vi "HelioLED.vi"() -> ()   [LabVIEW 2010]
uses:
  bricks/classes/DAQmxDigitalOut/DAQmxDigitalOut.lvclass
  bricks/classes/DAQmxAnalogOut/DAQmxAnalogOut/DAQmxAnalogOut.lvclass
panel:
  in  "period":dbl[unit]=20.0
  in  "startButton":bool
  in  "number of points":i32=1 min=1
  out "lower bound":dbl[unit]
  out "upper bound":dbl[unit]
  in  "setUpperBoundButton":bool
  in  "setLowerBoundButton":bool
  in  "doneButton":bool
  in  "voltage":dbl[unit](slide) scale=0.0..4.0
  in  "voltage source configuration":string(combo)
  in  "trigger configuration":string(combo)
  # "HelioLED"
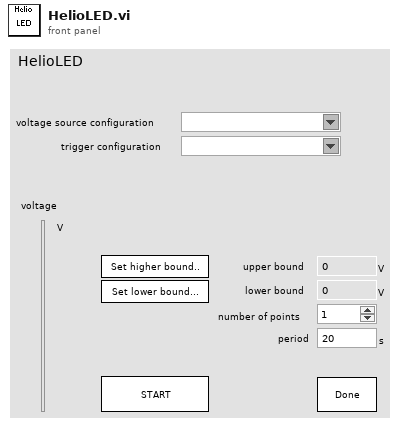
[diagram p1: front panel]
types:
  T1 = enum8{"Enabled", "Disabled", "Disabled and Grayed Out"}
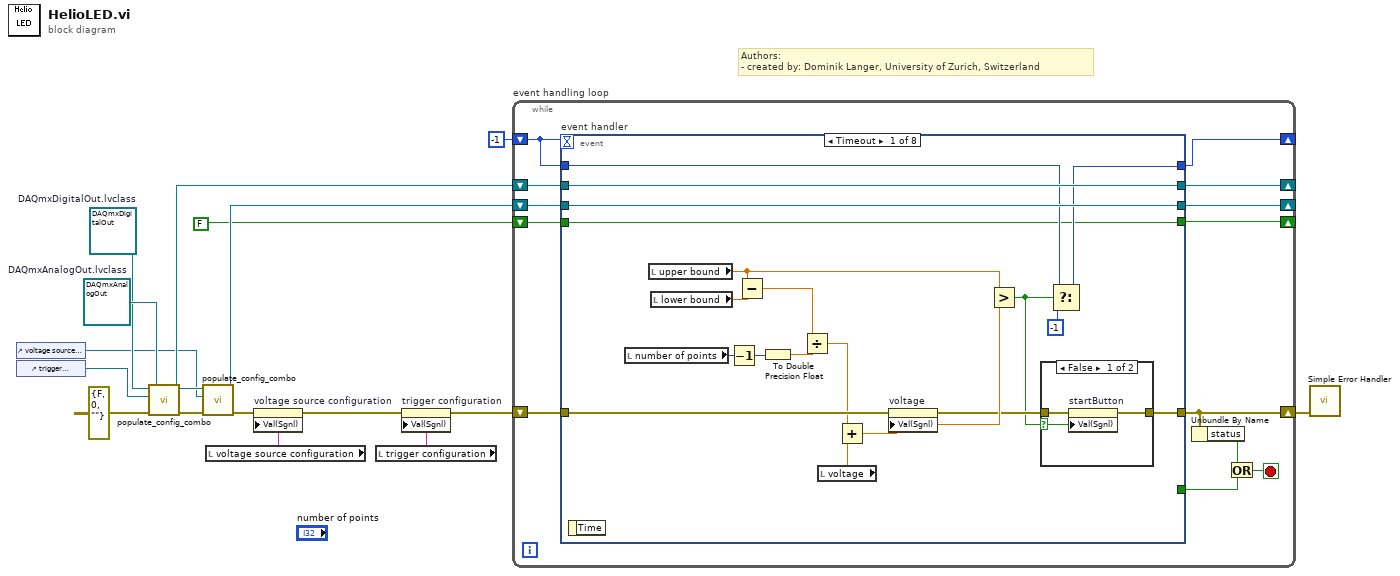
[diagram p0: block diagram]
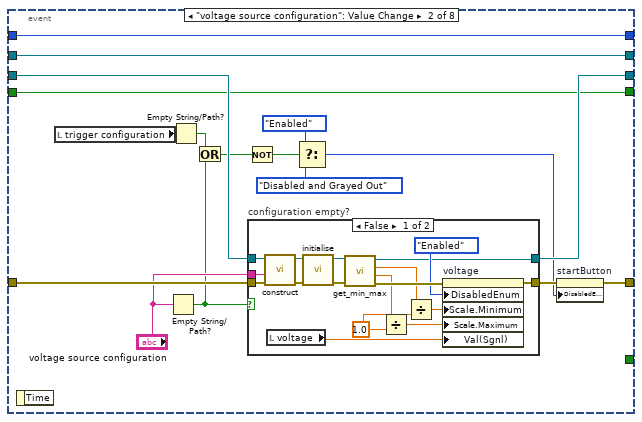
[diagram p3: hidden frame]
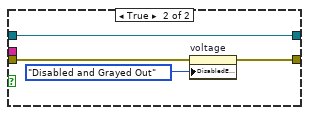
[diagram p4: hidden frame]
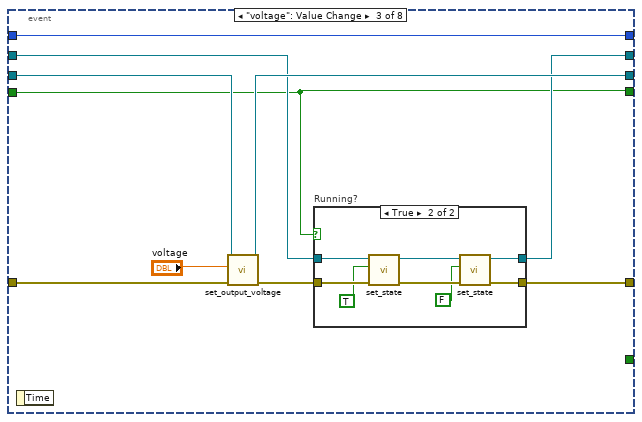
[diagram p5: hidden frame]
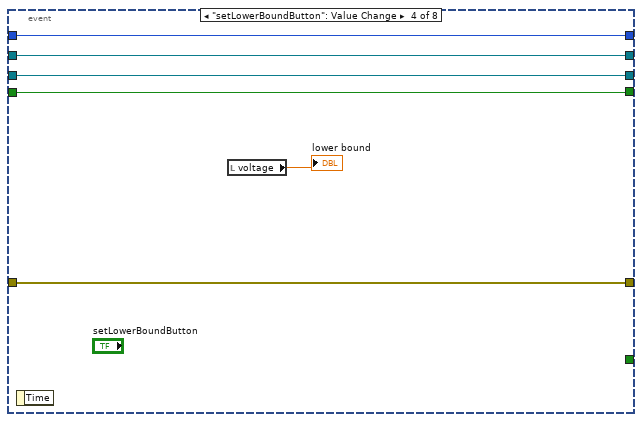
[diagram p7: hidden frame]
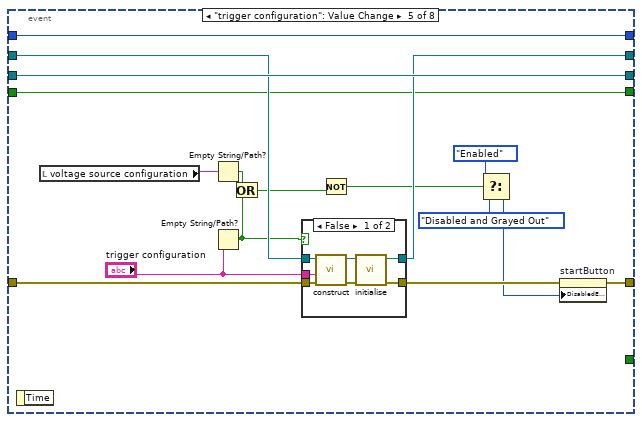
[diagram p8: hidden frame]
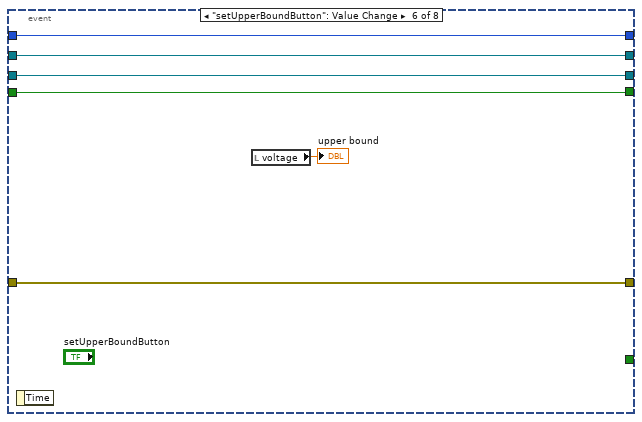
[diagram p10: hidden frame]
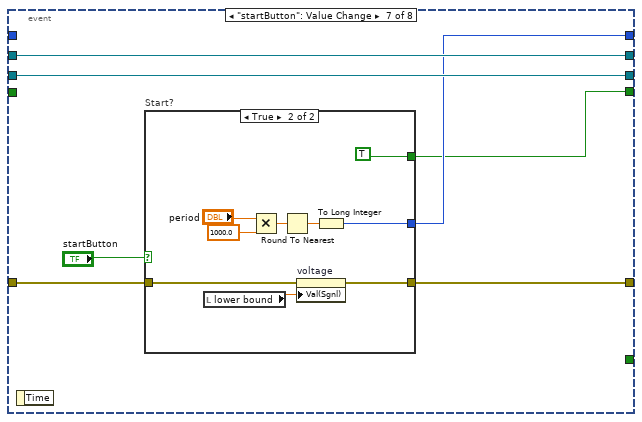
[diagram p11: hidden frame]
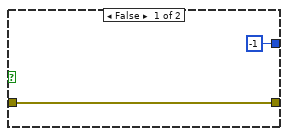
[diagram p12: hidden frame]
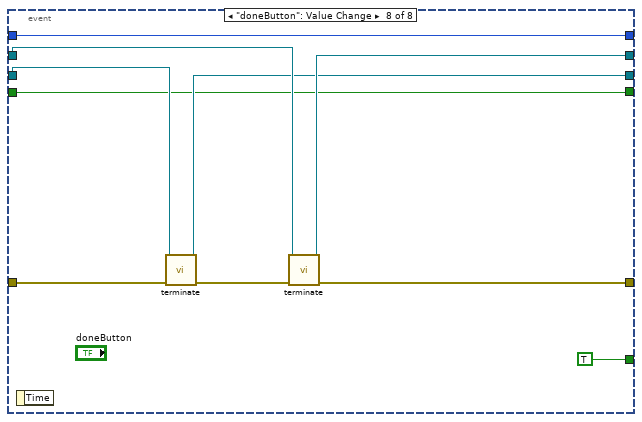
[diagram p13: hidden frame]
diagram:
  w14 = refnum<class "DAQmxAnalogOut.lvclass"> refnum  # DAQmxAnalogOut.lvclass
  w12 = refnum<class "DAQmxDigitalOut.lvclass"> refnum  # DAQmxDigitalOut.lvclass
  # "Authors: \n- created by: Dominik Langer, University of Zurich, Switzerland"
  n1 = control-ref of="voltage source configuration"() -> (w8:refnum<vi>)
  n2 = control-ref of="trigger configuration"() -> (w9:refnum<vi>)
  n3 = call-dynamic "populate_config_combo.vi"("error in (no error)"=errorcluster {"status"=FALSE, "code"=0, "source"=""}, "combo-box reference"=w9, "GenericPlugin in"=w12) -> ("error out"=w15:errorcluster, "GenericPlugin out"=w11:refnum<class "DAQmxDigitalOut.lvclass">)  [unwired: 7 in]
  n4 = call-dynamic "populate_config_combo.vi"("error in (no error)"=w15, "combo-box reference"=w8, "GenericPlugin in"=w14) -> ("error out"=w6:errorcluster, "GenericPlugin out"=w13:refnum<class "DAQmxAnalogOut.lvclass">)  [unwired: 7 in]
  n5 = local read "voltage source configuration"() -> (w3:string)
  n6 = property on="voltage source configuration" class="CmbBox"(error in=w6, "Val(Sgnl)"=w3) -> (error out=w5:errorcluster)  [unwired: 1 in, 1 out]
  n7 = local read "trigger configuration"() -> (w2:string)
  n8 = property on="trigger configuration" class="CmbBox"(error in=w5, "Val(Sgnl)"=w2) -> (error out=w4:errorcluster)  [unwired: 1 in, 1 out]
  n9 = while "event handling loop" {
    shift-right: [w28] -> _
    shift-left: -1 -> [w29]
    shift-right: [w26] -> w1
    shift-left: w4 -> [w27]
    shift-right: [w22] -> _
    shift-left: w11 -> [w20]
    shift-right: [w21] -> _
    shift-left: w13 -> [w19]
    shift-right: [w17] -> _
    shift-left: FALSE -> [w18]
    stop <- w23 stop-if-true
    n10 = event "event handler" shown="[0] Timeout" {
      selector: _ -> [_ _ _ _ _ _ _ _]
      dyn-events: _ -> [_ _ _ _ _ _ _ _]
      timeout: w29 -> [_ _ _ _ _ _ _ _]
      tunnel: [w34 w69 w100 w116 w133 w148 w153 w176] -> w28
      tunnel: w29 -> [w36 w69 w100 w116 w133 w148 _ w176]
      tunnel: w27 -> [w46 w67 w99 w115 w131 w147 w152 w169]
      tunnel: [w31 w59 w93 w115 w124 w147 w151 w168] -> w26
      tunnel: [_ _ _ _ _ _ _ TRUE] -> w25
      tunnel: [w48 w68 w92 w114 w129 w146 w155 w172] -> w22
      tunnel: [w47 w65 w96 w113 w132 w145 w154 w171] -> w21
      tunnel: w20 -> [w48 w68 w94 w114 w130 w146 w155 w173]
      tunnel: w19 -> [w47 w66 w97 w113 w132 w145 w154 w174]
      tunnel: [w33 w64 w91 w111 w128 w143 w150 w167] -> w17
      tunnel: w18 -> [w33 w64 w91 w111 w128 w143 _ w167]
      event Timeout {
        n11 = event-data() -> ()  [unwired: 1 in, 1 out]
        n12 = local read "number of points"() -> (w44:i32)
        n13 = local read "upper bound"() -> (w37:dbl[unit])
        n14 = local read "lower bound"() -> (w45:dbl[unit])
        n15 = Decrement(x=w44) -> (x-1=w43:i32)
        n16 = Subtract(x=w37, y=w45) -> (x-y=w42:dbl[unit])
        n17 = To Double Precision Float(number=w43) -> (double precision float=w41:dbl)
        n18 = Divide(x=w42, y=w41) -> (x/y=w39:dbl[unit])
        n19 = local read "voltage"() -> (w40:dbl[unit])
        n20 = Add(x=w39, y=w40) -> (x+y=w38:dbl[unit])
        n21 = property on="voltage" class="Slide (strict)"(error in=w46, "Val(Sgnl)"=w38) -> (error out=w32:errorcluster)  [unwired: 1 in, 1 out]
        n22 = Greater?(x=w37, y=w38) -> (0:w30:bool)
        n23 = case shown="False" w30 {
          selector: w30 -> [w49 _]
          tunnel: w32 -> [w51 w52]
          tunnel: [w50 w52] -> w31
          frame False {
            n24 = property on="startButton" class="Bool (strict)"(error in=w51, "Val(Sgnl)"=w49) -> (error out=w50:errorcluster)  [unwired: 1 in, 1 out]
          }
          frame True {
          }
        }
        n25 = Select(t=w36, s=w30, f=-1) -> (s? t:f=w34:i32)
      }
      event "voltage source configuration": Value Change {
        n26 = event-data() -> ()  [unwired: 1 in, 1 out]
        n27 = local read "trigger configuration"() -> (w62:string)
        n28 = Empty String/Path?(string/path="voltage source configuration") -> (empty?=w60:bool)
        n29 = Empty String/Path?(string/path=w62) -> (empty?=w61:bool)
        n30 = Or(x=w61, y=w60) -> (x .or. y?=w53:bool)
        n31 = Not(x=w53) -> (.not. x?=w54:bool)
        n32 = case "configuration empty?" shown="False" w60 {
          tunnel: w67 -> [w86 w89]
          tunnel: w66 -> [w85 w90]
          tunnel: [w81 w88] -> w58
          tunnel: [w71 w90] -> w65
          tunnel: "voltage source configuration" -> [w82 _]
          frame False {
            w72 = dbl[unit] 1.0 ("y")
            n33 = call-dynamic "construct.vi"("error in (no error)"=w86, "configuration name"=w82, "GenericPlugin in"=w85) -> ("error out"=w84:errorcluster, "GenericPlugin out"=w83:refnum<class "DAQmxAnalogOut.lvclass">)  [unwired: 7 in]
            n34 = local read "voltage"() -> (w70:dbl[unit])
            n35 = call-dynamic "initialise.vi"("error in (no error)"=w84, "DAQmxAnalogOut in"=w83) -> ("error out"=w80:errorcluster, "DAQmxAnalogOut out"=w79:refnum<class "DAQmxAnalogOut.lvclass">)  [unwired: 8 in]
            n36 = call "get_min_max.vi"("error in (no error)"=w80, "DAQmxAnalogOut.lvclass in"=w79) -> ("error out"=w78:errorcluster, "maximum"=w74:dbl[unit], "minimum"=w75:dbl[unit], "DAQmxAnalogOut.lvclass out"=w71:refnum<class "DAQmxAnalogOut.lvclass">)  [unwired: 6 in]
            n37 = Divide(x=w74, y=w72) -> (x/y=w73:dbl)
            n38 = Divide(x=w75, y=w72) -> (x/y=w76:dbl)
            n39 = property on="voltage" class="Slide (strict)"(error in=w78, "DisabledEnum"=T1."Enabled" ("Disabled"), "Scale.Minimum"=w76, "Scale.Maximum"=w73, "Val(Sgnl)"=w70) -> (error out=w81:errorcluster)  [unwired: 1 in, 1 out]
          }
          frame True {
            n40 = property on="voltage" class="Slide (strict)"(error in=w89, "DisabledEnum"=T1."Disabled and Grayed Out" ("Disabled")) -> (error out=w88:errorcluster)  [unwired: 1 in, 1 out]
          }
        }
        n41 = Select(t=T1."Enabled" ("Disabled"), s=w54, f=T1."Disabled and Grayed Out" ("Disabled")) -> (s? t:f=w55:T1)
        n42 = property on="startButton" class="Bool (strict)"(error in=w58, "DisabledEnum"=w55) -> (error out=w59:errorcluster)  [unwired: 1 in, 1 out]
      }
      event "voltage": Value Change {
        n43 = event-data() -> ()  [unwired: 1 in, 1 out]
        n44 = call "set_output_voltage.vi"("error in (no error)"=w99, "output value"="voltage", "DAQmxAnalogOut in"=w97) -> ("error out"=w95:errorcluster, "DAQmxAnalogOut out"=w96:refnum<class "DAQmxAnalogOut.lvclass">)  [unwired: 7 in]
        n45 = case "Running?" shown="True" w91 {
          tunnel: w95 -> [w101 w110]
          tunnel: w94 -> [w102 w109]
          tunnel: [w101 w106] -> w93
          tunnel: [w102 w104] -> w92
          frame False {
          }
          frame True {
            n46 = call "set_state.vi"("error in (no error)"=w110, "state"=TRUE, "DAQmxDigitalOut in"=w109) -> ("error out"=w107:errorcluster, "DAQmxDigitalOut out"=w105:refnum<class "DAQmxDigitalOut.lvclass">)  [unwired: 7 in]
            n47 = call "set_state.vi"("error in (no error)"=w107, "state"=FALSE, "DAQmxDigitalOut in"=w105) -> ("error out"=w106:errorcluster, "DAQmxDigitalOut out"=w104:refnum<class "DAQmxDigitalOut.lvclass">)  [unwired: 7 in]
          }
        }
      }
      event "setLowerBoundButton": Value Change {
        n48 = event-data() -> ()  [unwired: 1 in, 1 out]
        n49 = local read "voltage"() -> (→"lower bound":dbl[unit])
      }
      event "trigger configuration": Value Change {
        n50 = event-data() -> ()  [unwired: 1 in, 1 out]
        n51 = local read "voltage source configuration"() -> (w127:string)
        n52 = Empty String/Path?(string/path=w127) -> (empty?=w120:bool)
        n53 = Empty String/Path?(string/path="trigger configuration") -> (empty?=w117:bool)
        n54 = Or(x=w120, y=w117) -> (x .or. y?=w119:bool)
        n55 = case shown="False" w117 {
          tunnel: w131 -> [w138 w142]
          tunnel: w130 -> [w137 w141]
          tunnel: [w136 w141] -> w129
          tunnel: "trigger configuration" -> [w135 _]
          tunnel: [w134 w142] -> w125
          frame False {
            n56 = call-dynamic "construct.vi"("error in (no error)"=w138, "configuration name"=w135, "GenericPlugin in"=w137) -> ("error out"=w140:errorcluster, "GenericPlugin out"=w139:refnum<class "DAQmxDigitalOut.lvclass">)  [unwired: 7 in]
            n57 = call-dynamic "initialise.vi"("error in (no error)"=w140, "DAQmxDigitalOut in"=w139) -> ("error out"=w134:errorcluster, "DAQmxDigitalOut out"=w136:refnum<class "DAQmxDigitalOut.lvclass">)  [unwired: 8 in]
          }
          frame True {
          }
        }
        n58 = Not(x=w119) -> (.not. x?=w118:bool)
        n59 = Select(t=T1."Enabled" ("Disabled"), s=w118, f=T1."Disabled and Grayed Out" ("Disabled")) -> (s? t:f=w121:T1)
        n60 = property on="startButton" class="Bool (strict)"(error in=w125, "DisabledEnum"=w121) -> (error out=w124:errorcluster)  [unwired: 1 in, 1 out]
      }
      event "setUpperBoundButton": Value Change {
        n61 = event-data() -> ()  [unwired: 1 in, 1 out]
        n62 = local read "voltage"() -> (→"upper bound":dbl[unit])
      }
      event "startButton": Value Change {
        n63 = event-data() -> ()  [unwired: 1 in, 1 out]
        n64 = case "Start?" shown="True" "startButton" {
          tunnel: [-1 w162] -> w153
          tunnel: w152 -> [w157 w161]
          tunnel: [w157 w160] -> w151
          tunnel: [_ TRUE] -> w150
          frame False {
          }
          frame True {
            n65 = local read "lower bound"() -> (w159:dbl[unit])
            n66 = Multiply(x="period", y=dbl[unit] 1000.0) -> (x*y=w164:dbl)
            n67 = Round To Nearest(number=w164) -> (nearest integer value=w163:dbl)
            n68 = property on="voltage" class="Slide (strict)"(error in=w161, "Val(Sgnl)"=w159) -> (error out=w160:errorcluster)  [unwired: 1 in, 1 out]
            n69 = To Long Integer(number=w163) -> (32bit integer=w162:i32)
          }
        }
      }
      event "doneButton": Value Change {
        n70 = event-data() -> ()  [unwired: 1 in, 1 out]
        n71 = call-dynamic "terminate.vi"("error in (no error)"=w169, "DAQmxAnalogOut in"=w174) -> ("error out"=w170:errorcluster, "DAQmxAnalogOut out"=w171:refnum<class "DAQmxAnalogOut.lvclass">)  [unwired: 8 in]
        n72 = call-dynamic "terminate.vi"("error in (no error)"=w170, "DAQmxDigitalOut in"=w173) -> ("error out"=w168:errorcluster, "DAQmxDigitalOut out"=w172:refnum<class "DAQmxDigitalOut.lvclass">)  [unwired: 8 in]
      }
    }
    n73 = Unbundle By Name(w26) -> ("status"=w24:bool)
    n74 = Or(x=w24, y=w25) -> (x .or. y?=w23:bool)
  }
  n75 = call <vilib>:"Simple Error Handler.vi"("error in (no error)"=w1) -> ()  [unwired: 4 in, 5 out]
